vi "wholeBrainImagerGreenBlue.vi"() -> ()   [LabVIEW 2017]
uses:
  globalDevices.vi
panel:
  in  "mode":u16(ring) items=["Green", "Blue"]
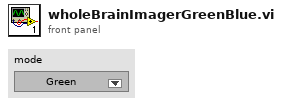
[diagram p1: front panel]
types:
  T1 = cluster{"serialPort":refnum<visa-resource-name>, "error":errorcluster, "power (mW)":dbl, "wavelength (nm)":dbl, "type":string, "shutter":i32}[]
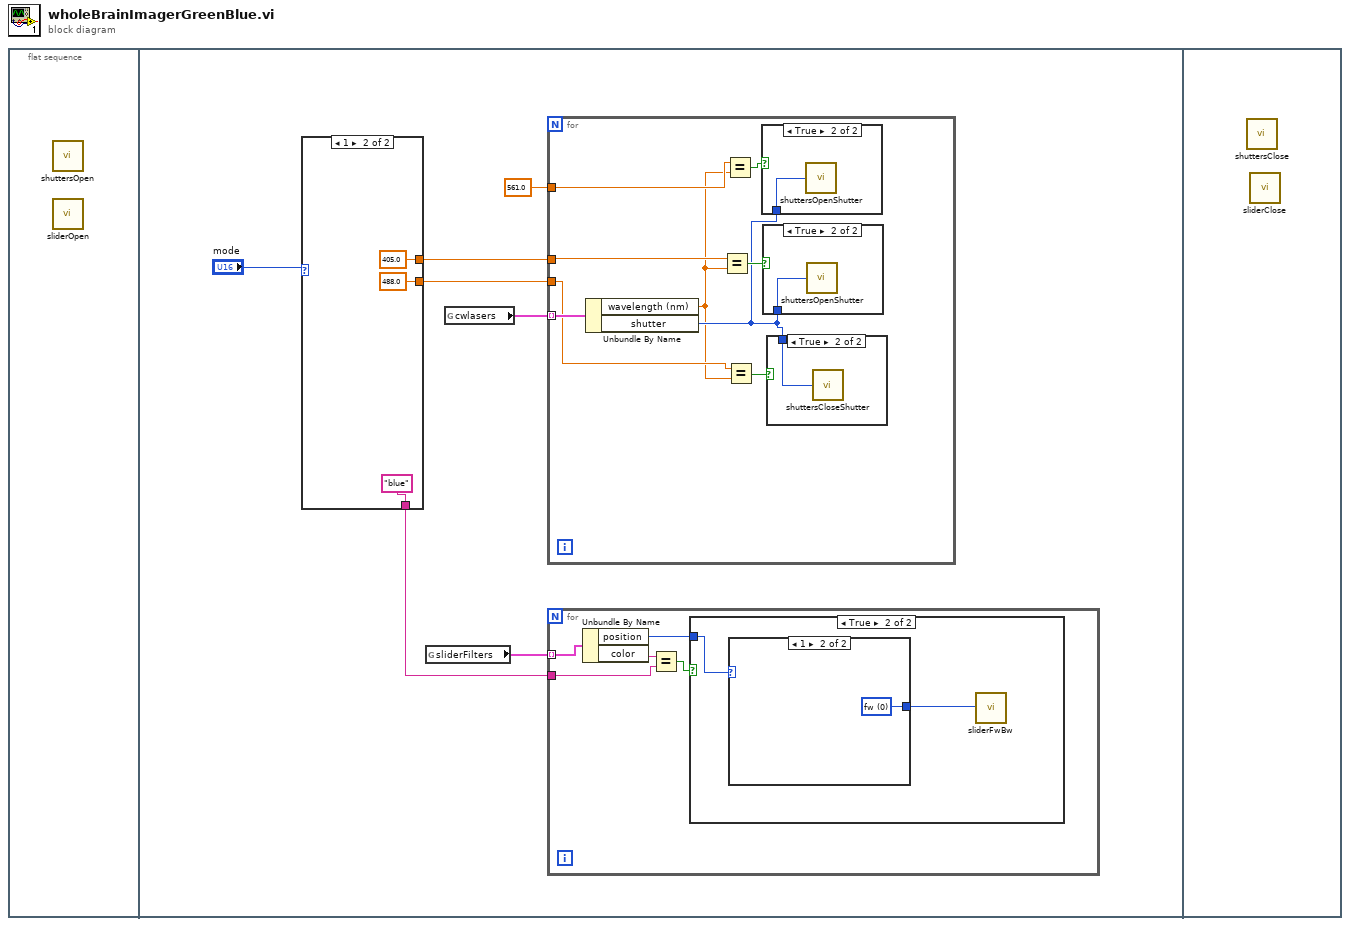
[diagram p0: block diagram]
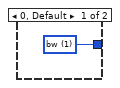
[diagram p3: hidden frame]
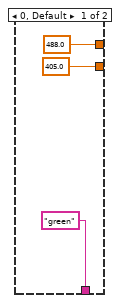
[diagram p7: hidden frame]
diagram:
  n1 = flat-sequence {
    frame #0 {
      n2 = call "shuttersOpen.vi"() -> ()  [unwired: 12 in]
      n3 = call "sliderOpen.vi"() -> ()  [unwired: 2 in, 1 out]
    }
    frame #1 {
      n4 = case shown="1" "mode" {
        tunnel: [488.0 405.0] -> w5
        tunnel: [405.0 488.0] -> w4
        tunnel: ["green" "blue"] -> w3
        frame 0, Default {
        }
        frame 1 {
        }
      }
      n5 = global read "globalDevices.vi" "sliderFilters"() -> (w1:cluster{"position":u16, "color":string}[])
      n6 = global read "globalDevices.vi" "cwlasers"() -> (w6:T1)
      n7 = for {
        tunnel: w6 -> [w25] mode=indexing
        tunnel: w5 -> [w24]
        tunnel: w4 -> [w22]
        tunnel: 561.0 -> [w18]
        n8 = Unbundle By Name(w25) -> ("wavelength (nm)"=w17:dbl, "shutter"=w20:i32)
        n9 = Equal?(x=w24, y=w17) -> (x = y?=w23:bool)
        n10 = Equal?(x=w18, y=w17) -> (x = y?=w19:bool)
        n11 = Equal?(x=w22, y=w17) -> (x = y?=w21:bool)
        n12 = case shown="True" w19 {
          tunnel: w20 -> [_ w26]
          frame False {
          }
          frame True {
            n13 = call "shuttersOpenShutter.vi"("shutter"=w26) -> ()  [unwired: 1 in]
          }
        }
        n14 = case shown="True" w23 {
          tunnel: w20 -> [_ w28]
          frame False {
          }
          frame True {
            n15 = call "shuttersOpenShutter.vi"("shutter"=w28) -> ()  [unwired: 1 in]
          }
        }
        n16 = case shown="True" w21 {
          tunnel: w20 -> [_ w27]
          frame False {
          }
          frame True {
            n17 = call "shuttersCloseShutter.vi"("shutter"=w27) -> ()  [unwired: 1 in]
          }
        }
      }
      n18 = for {
        tunnel: w1 -> [w12] mode=indexing
        tunnel: w3 -> [w10]
        n19 = Unbundle By Name(w12) -> ("position"=w9:u16, "color"=w11:string)
        n20 = Equal?(x=w11, y=w10) -> (x = y?=w8:bool)
        n21 = case shown="True" w8 {
          tunnel: w9 -> [_ w14]
          frame False {
          }
          frame True {
            n22 = case shown="1" w14 {
              tunnel: [w15 w16] -> w13
              frame 0, Default {
                w15 = u16 1 items=["fw", "bw"] ("mode")
              }
              frame 1 {
                w16 = u16 0 items=["fw", "bw"] ("mode")
              }
            }
            n23 = call "sliderFwBw.vi"("mode"=w13) -> ()  [unwired: 1 in]
          }
        }
      }
    }
    frame #2 {
      n24 = call "shuttersClose.vi"() -> ()  [unwired: 12 in]
      n25 = call "sliderClose.vi"() -> ()  [unwired: 2 in, 1 out]
    }
  }
